vi "Flash_ADB.vi"(11 "Flash Bat File":string="adb_flash.bat") -> (0 "error out":errorcluster, 1 "standard output":string, 2 "return code":i32, 3 "Result":bool)   [LabVIEW 2018]
panel:
  out "cmd line":string
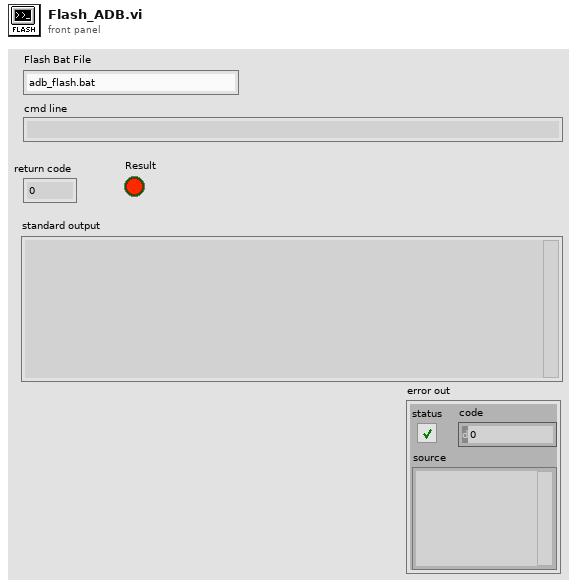
[diagram p1: front panel]
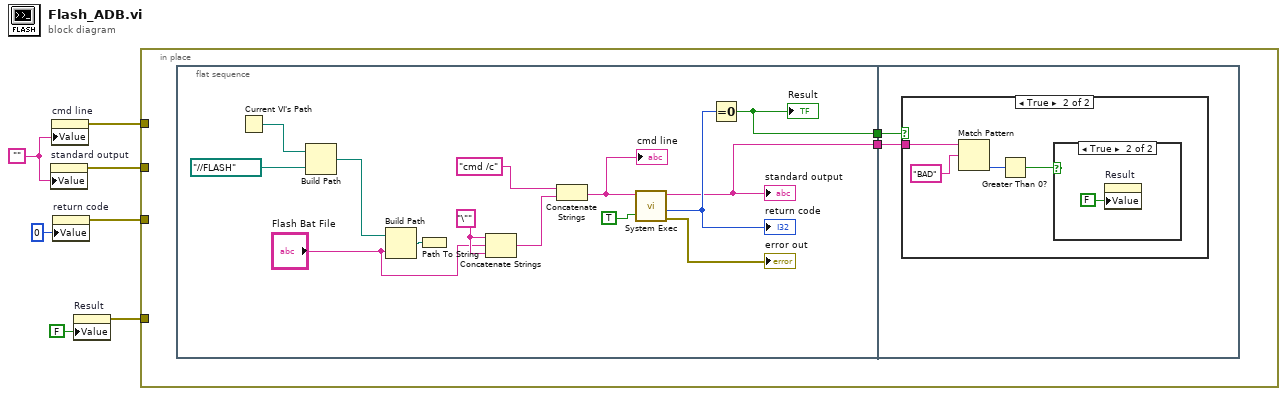
[diagram p0: block diagram]
diagram:
  w3 = ""
  n1 = property on="standard output" class="Str"("Value"=w3) -> (error out=w4:errorcluster)  [unwired: 2 in, 1 out]
  n2 = property on="cmd line" class="Str"("Value"=w3) -> (error out=w5:errorcluster)  [unwired: 2 in, 1 out]
  n3 = property on="return code" class="DigNum (strict)"("Value"=0 ("return code")) -> (error out=w2:errorcluster)  [unwired: 2 in, 1 out]
  n4 = property on="Result" class="Bool (strict)"("Value"=FALSE ("Result")) -> (error out=w7:errorcluster)  [unwired: 2 in, 1 out]
  n5 = in-place {
    in-place-border: w7 -> [_]
    in-place-border: w5 -> [_]
    in-place-border: w4 -> [_]
    in-place-border: w2 -> [_]
    n6 = flat-sequence {
      tunnel: [w16] -> w9
      tunnel: [w15] -> w8
      tunnel: w9 -> [w25]
      tunnel: w8 -> [w24]
      frame #0 {
        w20 = "\"" ("string")
        n7 = Current VI's Path() -> (path=w13:path)
        n8 = Build Path(base path=w13, name or relative path=path "../../FLASH") -> (appended path=w11:path)
        n9 = Build Path(base path=w11, name or relative path="Flash Bat File") -> (appended path=w21:path)
        n10 = Path To String(path=w21) -> ()  [unwired: 1 out]
        n11 = Concatenate Strings(w20, "Flash Bat File", w20) -> (w14:string)
        n12 = Concatenate Strings("cmd /c" ("string"), w14) -> (w18:string)
        "cmd line" <- w18
        n13 = call <vilib>:"System Exec.vi"("run minimized? (F)"=TRUE, "command line"=w18) -> ("error out"=→"error out":errorcluster, "return code"=w22:i32, "standard output"=w15:string)  [unwired: 6 in, 1 out]
        "return code" <- w22
        "standard output" <- w15
        n14 = Equal To 0?(x=w22) -> (x = 0?=w16:bool)
        "Result" <- w16
      }
      frame #1 {
        n15 = case shown="True" w25 {
          tunnel: w24 -> [_ w29]
          frame False {
          }
          frame True {
            n16 = Match Pattern(string=w29, regular expression="BAD") -> (offset past match=w27:i32)  [unwired: 1 in, 3 out]
            n17 = Greater Than 0?(x=w27) -> (x > 0?=w26:bool)
            n18 = case shown="True" w26 {
              frame False {
              }
              frame True {
                n19 = property on="Result" class="Bool (strict)"("Value"=FALSE ("Result")) -> ()  [unwired: 2 in, 2 out]
              }
            }
          }
        }
      }
    }
  }
